vi "Client.vi"() -> ()   [LabVIEW 2019]
uses:
  <vilib>/httpClient/PUTBuffer.vi
  <vilib>/httpClient/LabVIEWHTTPClient.lvlib
panel:
  in  "stop":bool
  in  "Remote Light":bool
  out "body":string
  out "headers":string
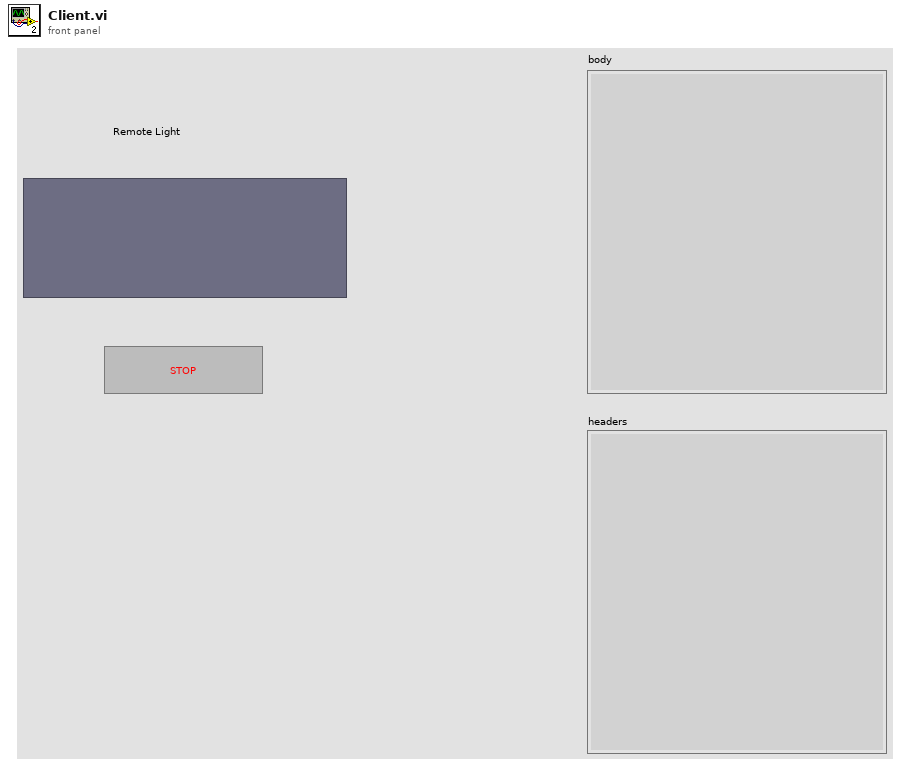
[diagram p1: front panel]
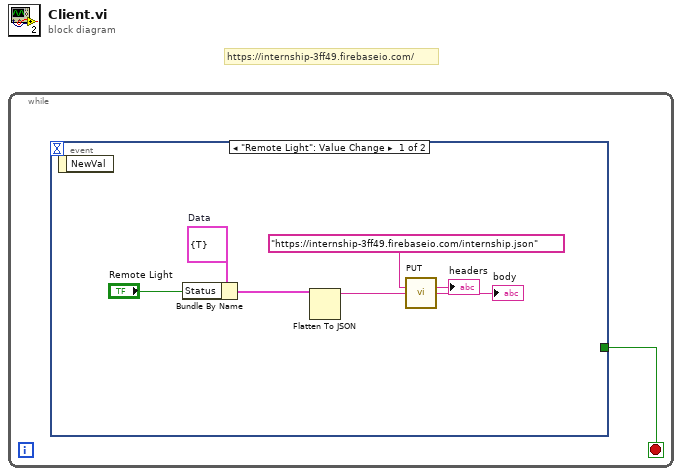
[diagram p0: block diagram]
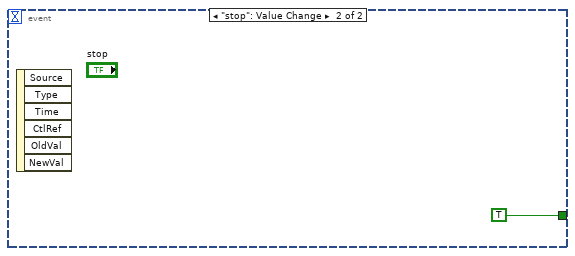
[diagram p2: hidden frame]
diagram:
  # "https://internship-3ff49.firebaseio.com/"
  n1 = while {
    stop <- w1 stop-if-true
    n2 = event shown="[0] \"Remote Light\": Value Change" {
      selector: _ -> [_ _]
      dyn-events: _ -> [_ _]
      timeout: _ -> [_ _]
      tunnel: [_ TRUE] -> w1
      event "Remote Light": Value Change {
        w4 = cluster{"Status":bool} {"Status"=TRUE}  # Data
        n3 = event-data() -> ()  [unwired: 1 in, 1 out]
        n4 = Bundle By Name(cluster=w4, "Status"="Remote Light") -> (w2:cluster{"Status":bool})
        n5 = Flatten To JSON(anything=w2) -> (JSON string=w7:string)  [unwired: 2 in, 1 out]
        n6 = call-poly <vilib>:"PUT.vi"("url"="https://internship-3ff49.firebaseio.com/internship.json", "buffer"=w7) -> ("headers"=→"headers":string, "body"=→"body":string)  [unwired: 10 in, 2 out]
      }
      event "stop": Value Change {
        n7 = event-data() -> ()  [unwired: 1 in, 6 out]
      }
    }
  }
